vi "Publisher Do.vi"(8 "error in (no error)":errorcluster, 10 "Publisher in":refnum<class "Publisher.lvclass">, 11 "Subscribe Msg":refnum<class "Instrument Sequencer Sender Msg.lvclass">) -> (0 "error out":errorcluster, 2 "Publisher out":refnum<class "Publisher.lvclass">)   [LabVIEW 2020, in "Instrument Handler.lvlib" / "Instrument Sequencer Sender Msg.lvclass"]
doc: "This VI delivers the message to the actor by calling the appropriate method(s) on the actor.\n\nThis implementation drops messages by default."
uses:
  Instrument Sequencer Sender Msg.lvclass
  PPL/HDH.Actor Framework.Core.Publisher.lvlibp/Publisher/Publisher.lvclass
  PPL/HDH.Actor Framework.Core.Publisher.lvlibp/Publisher Messages/Sender Msg/Sender Msg.lvclass
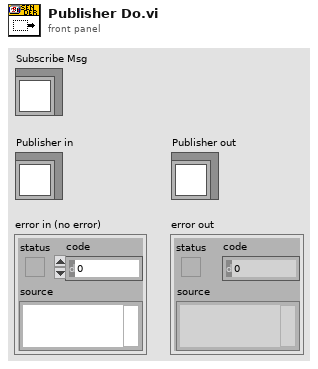
[diagram p1: front panel]
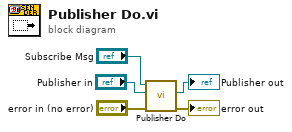
[diagram p0: block diagram]
diagram:
  n1 = call-parent "Publisher Do.vi"("error in (no error)"="error in (no error)", "Publisher in"="Publisher in", "Subscribe Msg"="Subscribe Msg") -> ("error out"=→"error out":errorcluster, "Publisher out"=→"Publisher out":refnum<class "Publisher.lvclass">)  [unwired: 7 in]
